vi "Asylum_Driver_XYMetersToVoltageArray.vi"(8 "error in (no error)":errorcluster, 9 "Y Coordinate":dbl[](array[numeric]), 10 "X Coordinate":dbl[](array[numeric]), 11 "Application":refnum<k7>) -> (0 "error out":errorcluster, 1 "Y Voltage":dbl[](array[numeric]), 2 "X Voltage":dbl[](array[numeric]), 3 "Application":refnum<k7>)   [LabVIEW 2019]
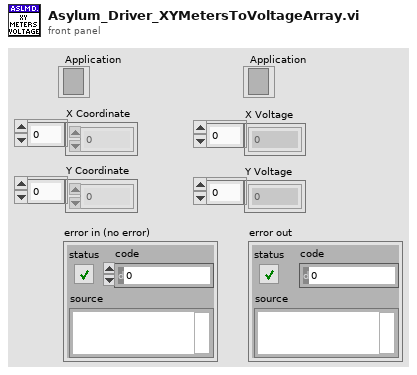
[diagram p1: front panel]
types:
  T1 = cluster{"XLVDT Sens":dbl, "YLVDT Sens":dbl, "XLVDT Offset":dbl, "YLVDT Offset":dbl}
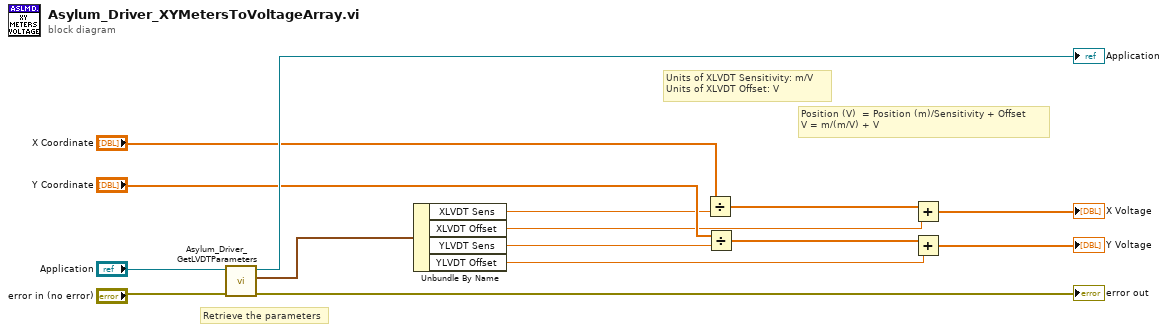
[diagram p0: block diagram]
diagram:
  # "Retrieve the parameters"
  # "Units of XLVDT Sensitivity: m/V\nUnits of XLVDT Offset: V"
  # "Position (V)  = Position (m)/Sensitivity + Offset\nV = m/(m/V) + V"
  n1 = call "Asylum_Driver_GetLVDTParameters.vi"("error in (no error)"="error in (no error)", "Application"="Application") -> ("error out"=→"error out":errorcluster, "LVDT Parameters"=w7:T1, "Application"=→"Application":refnum<k7>)  [unwired: 7 in]
  n2 = Unbundle By Name(w7) -> ("XLVDT Sens"=w4:dbl, "XLVDT Offset"=w1:dbl, "YLVDT Sens"=w5:dbl, "YLVDT Offset"=w2:dbl)
  n3 = Divide(x="X Coordinate", y=w4) -> (x/y=w3:dbl[])
  n4 = Divide(x="Y Coordinate", y=w5) -> (x/y=w6:dbl[])
  n5 = Add(x=w3, y=w1) -> (x+y=→"X Voltage":dbl[])
  n6 = Add(x=w6, y=w2) -> (x+y=→"Y Voltage":dbl[])
